vi "LIDAR V3 Mem1 Manager.vi"(0 "MeanFIFO":refnum<k21>="MeanVals1", 3 "StartAlgo":refnum<k21>="StartAlg2", 5 "MemRequest":refnum<k21>="MemRequest1", 6 "SignalMem":refnum<k21>="SignalMem1", 7 "MemDataAi":refnum<k21>="MemDataAi1", 8 "MemRequestDeb":refnum<k21>="MemRequestDeb1", 9 "MemDataDeb":refnum<k21>="MemDataDeb1", 10 "MemData":refnum<k21>="MemData1", 11 "Source Clk":refnum<k21>="100 MHz Clock") -> ()   [LabVIEW 2015]
uses:
  <vilib>/Platform/TimedLoop/XDataNode/timing_clust.ctl
  <vilib>/Platform/TimedLoop/XDataNode/nitl_modes.ctl
  <vilib>/Platform/TimedLoop/XDataNode/wakeup.ctl
  <vilib>/rvi/Emulation/niFpgaSctlEmulationGetInTimedLoop.vi
  <vilib>/rvi/Emulation/niFpgaEmulationReportErrorSimple.vi
  <vilib>/rvi/Emulation/niFpgaGetClockAttributes.vi
  <vilib>/rvi/Emulation/niFpgaCriticalErrorInLSC.vi
  <vilib>/rvi/DataTransferAndStorage/Container/Common/niFpgaContainerExecOnDevCompGetState.vi
  <vilib>/rvi/Emulation/niFpgaEmulationIsFPGAContextNoSignature.vi
  <vilib>/rvi/DataTransferAndStorage/Container/Common/niFpgaContainerGetUniqueNameForEmu.vi
  <vilib>/rvi/Emulation/niFpgaProcessEmulError.vi
  <vilib>/rvi/errors/nirviReportUnexpectedCaseInternalError (U32).vi
  <vilib>/rvi/Memory/Memory_Emulation/niFpgaMemoryEmulationCacheClearOnFirstRun.vi
  <vilib>/rvi/Memory/Memory_Emulation/nirvimemoryEmulationManagerCache_MakeExclusive.vi
  <vilib>/rvi/Memory/Memory_Emulation/niFpgaMemoryEmulationValidateCache.vi
  <vilib>/rvi/Memory/Memory_Emulation/nirvimemoryEmulationManagerCache_InsertValue.vi
  <vilib>/Utility/error.llb/Clear Errors.vi
  <vilib>/rvi/Memory/Memory_Emulation/nirvimemoryEmulationManagerCache_ReleaseExclusive.vi
  <vilib>/rvi/Memory/Memory_Emulation/nirvimemoryEmulationManagerCache_GetValue.vi
  <vilib>/rvi/Memory/Memory_Emulation/nirvimemoryEmulationManagerCache_SetValue.vi
  <vilib>/rvi/Emulation/niFpgaSctlEmulationResourceMgr.vi
  <vilib>/rvi/errors/niFpgaSetErrorForExecOnDevCompSimple.vi
  <vilib>/rvi/eio/common/nirviEmuReportErrorAndStop.vi
  <vilib>/rvi/FIFO/Fifo_Resource/nirvififoEmulationSetSize.vi
  <vilib>/rvi/FIFO/Fifo_Resource/nirviFifoEmulationQueueMgr.vi
  <instcachedir>/0/nirviFifoEmulationQueueMgr_E5CAEC123FF24DC58D834DCA3CDAA9B5.lvgen/nirviFifoEmulationQueueMgr_E5CAEC123FF24DC58D834DCA3CDAA9B5_002.vi
  <vilib>/rvi/FIFO/Fifo_Resource/nirvififoEmulationDetermineInputValidOut.vi
  <vilib>/rvi/FIFO/Fifo_Resource/nirvififoEmulationCreateLock.vi
  <vilib>/rvi/FIFO/Fifo_Resource/nirvififoEmulationObtainLock.vi
  <vilib>/rvi/FIFO/Fifo_Resource/nirvififoEmulationReleaseLock.vi
  <vilib>/rvi/occurrence/nirviWaitOnOccurrenceBase.vi
  <vilib>/rvi/errors/nirviReportUnexpectedCaseInternalError.vi
  <vilib>/rvi/interface/RandomDataEmulation/niFpgaRandomDataHandleErrors.vi
  <instcachedir>/0/nirviFifoEmulationQueueMgr_E5CAEC123FF24DC58D834DCA3CDAA9B5.lvgen/nirviFifoEmulationQueueMgr_E5CAEC123FF24DC58D834DCA3CDAA9B5_001.vi
  <vilib>/Platform/TimedLoop/XDataNode/XDataNode.xnode
  <vilib>/rvi/FXPMathLib/FxpAdd/XNode/nifxpmath_Add.xnode
  <vilib>/rvi/DataTransferAndStorage/Container/XNode/niFpgaContainer.xnode
  <vilib>/rvi/Memory/Memory_Emulation/niFpgaMemoryEmulationRefIn.vi
  <vilib>/rvi/FIFO/Fifo_Resource/niFpgaFifoEmulationRefIn.vi
  <vilib>/Platform/TimedLoop/XDataNode/XDNodeRunTimeDep.lvlib
  <vilib>/rvi/FXPMathLib/sim/FxpSim.dll
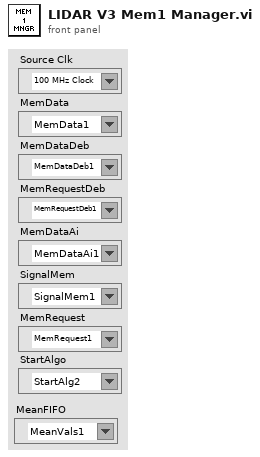
[diagram p1: front panel]
types:
  T1 = typedef "XDNodeRunTimeDep.lvlib/timing_clust.ctl" = cluster{"Expected End [f-1]":u64, "Actual End [f-1]":u64, "Finished Late? [f-1]":bool, "Expected End [i-1]":u64, "Actual End [i-1]":u64, "Finished Late? [i-1]":bool, "Expected Start [i]":u64, "Actual Start [i]":u64, "Expected Start [f]":u64, "Actual Start [f]":u64, "Source Name":string, "Structure Name":string, "Period":i64, "Deadline":i64, "Offset":i64, "Start":i64, "Priority":i32, "Timeout":i32, "Mode":T2, "Wakeup Reason":T3, "Error":errorcluster, "Source Type":string, "Secondary Source Type":string, "Global End Time":u64, "Global Start Time":u64, "Frame Duration":u64, "Iteration Duration":u64, "Assigned CPU":i32, "I/O Scan Engine Mode":u32}
  T2 = typedef "XDNodeRunTimeDep.lvlib/nitl_modes.ctl" = enum32{"No Change", "Process missed periods, maintain original phase", "Discard missed periods, maintain original phase", "Process missed periods, ignore original phase", "Discard missed periods, ignore original phase"}
  T3 = typedef "XDNodeRunTimeDep.lvlib/wakeup.ctl" = enum32{"Normal", "Aborted", "Asynchronous wakeup", "Timing source error", "Timed loop error", "Timeout"}
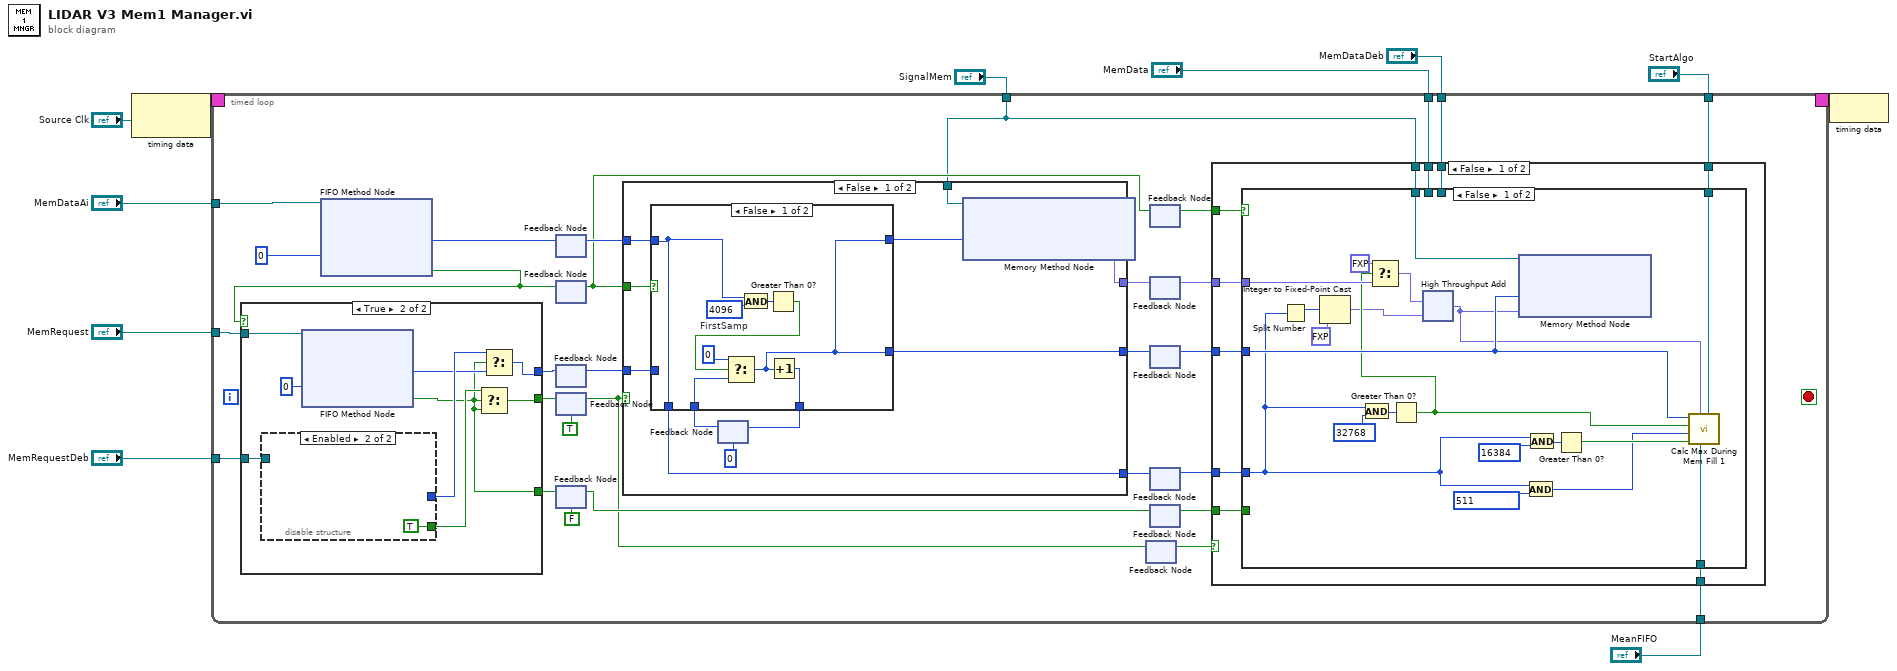
[diagram p0: block diagram]
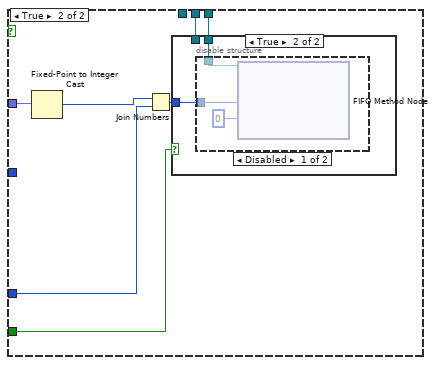
[diagram p2: hidden frame]
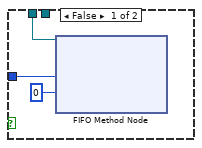
[diagram p3: hidden frame]
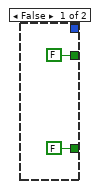
[diagram p8: hidden frame]
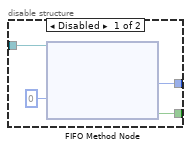
[diagram p9: hidden frame]
diagram:
  n1 = node-c288("Source Clk") -> (w11:T1)
  n2 = timed-loop {
    timing: w11 -> [_]
    timing-out: [_] -> w10
    tunnel: "MemDataAi" -> [w29]
    tunnel: "MemRequest" -> [w28]
    tunnel: "MemRequestDeb" -> [w27]
    tunnel: "SignalMem" -> [w26]
    tunnel: "MemData" -> [w25]
    tunnel: "MemDataDeb" -> [w24]
    tunnel: "MeanFIFO" -> [w13]
    tunnel: "StartAlgo" -> [w12]
    stop <- _ stop-if-true
    n3 = xnode ("FIFO Method Node")("Timeout"=0, "FIFO In"=w29) -> ("Element"=w41:u32, "Timed Out?"=w38:bool)  [unwired: 1 out]
    n4 = case shown="True" w38 {
      tunnel: [FALSE ("Timed Out?") w116] -> w39
      tunnel: [_ w113] -> w37
      tunnel: [FALSE ("Timed Out?") w112] -> w32
      tunnel: w28 -> [_ w111]
      tunnel: w27 -> [_ w110]
      frame False {
      }
      frame True {
        n5 = disable-structure shown="Enabled" {
          disable-tunnel: [w121 TRUE ("Timed Out?")] -> w117
          disable-tunnel: [w120 _] -> w115
          disable-tunnel: w110 -> [w119 _]
          frame Disabled {
            n6 = xnode ("FIFO Method Node")("Timeout"=0, "FIFO In"=w119) -> ("Element"=w120:u32, "Timed Out?"=w121:bool)  [unwired: 1 out]
          }
          frame Enabled {
          }
        }
        n7 = xnode ("FIFO Method Node")("Timeout"=0, "FIFO In"=w111) -> ("Element"=w114:u32, "Timed Out?"=w112:bool)  [unwired: 1 out]
        n8 = Select(t=w117, s=w112, f=w112) -> (s? t:f=w116:bool)
        n9 = Select(t=w115, s=w112, f=w114) -> (s? t:f=w113:u32)
      }
    }
    n10 = feedback-in #1(w41) -> ()
    n11 = feedback #1() -> (w36:u32)  [unwired: 1 in]
    n12 = feedback-in #2(w38) -> ()
    n13 = feedback #2() -> (w35:bool)  [unwired: 1 in]
    n14 = feedback-in #3(w37) -> ()
    n15 = feedback #3() -> (w34:u32)  [unwired: 1 in]
    n16 = feedback-in #4(w39) -> ()
    n17 = feedback #4(TRUE ("Timed Out?")) -> (w15:bool)
    n18 = feedback-in #5(w32) -> ()
    n19 = feedback #5(FALSE ("Timed Out?")) -> (w33:bool)
    n20 = case shown="False" w15 {
      tunnel: w36 -> [w97 _]
      tunnel: w35 -> [w96 _]
      tunnel: w34 -> [w95 _]
      tunnel: w26 -> [w94 _]
      tunnel: [w93 _] -> w23
      tunnel: [w91 _] -> w22
      tunnel: [w87 _] -> w21
      frame False {
        n21 = feedback #6(u32 0 ("Element")) -> (w88:u32)
        n22 = case shown="False" w96 {
          tunnel: w97 -> [w104 _]
          tunnel: [w98 w107] -> w92
          tunnel: w95 -> [_ w107]
          tunnel: [w104 w107] -> w91
          tunnel: [w99 w106] -> w89
          tunnel: w88 -> [w100 w106]
          tunnel: [w98 w106] -> w87
          frame False {
            w105 = u32 4096  # FirstSamp
            n23 = And(x=w104, y=w105) -> (x .and. y?=w103:u32)
            n24 = Greater Than 0?(x=w103) -> (x > 0?=w102:bool)
            n25 = Select(t=u32 0 ("Element"), s=w102, f=w100) -> (s? t:f=w98:u32)
            n26 = Increment(x=w98) -> (x+1=w99:u32)
          }
          frame True {
          }
        }
        n27 = feedback-in #6(w89) -> ()
        n28 = xnode ("Memory Method Node")("Address"=w92, "Memory In"=w94) -> ("Data"=w93:fxp<+/-,22,22>)  [unwired: 1 out]
      }
      frame True {
      }
    }
    n29 = feedback-in #7(w15) -> ()
    n30 = feedback #7() -> (w14:bool)  [unwired: 1 in]
    n31 = feedback-in #8(w35) -> ()
    n32 = feedback #8() -> (w20:bool)  [unwired: 1 in]
    n33 = feedback-in #9(w23) -> ()
    n34 = feedback #9() -> (w19:fxp<+/-,22,22>)  [unwired: 1 in]
    n35 = feedback-in #10(w21) -> ()
    n36 = feedback #10() -> (w18:u32)  [unwired: 1 in]
    n37 = feedback-in #11(w22) -> ()
    n38 = feedback #11() -> (w17:u32)  [unwired: 1 in]
    n39 = feedback-in #12(w33) -> ()
    n40 = feedback #12() -> (w16:bool)  [unwired: 1 in]
    n41 = case shown="False" w14 {
      tunnel: w26 -> [w51 _]
      tunnel: w25 -> [w50 _]
      tunnel: w24 -> [w49 _]
      tunnel: w20 -> [w48 _]
      tunnel: w19 -> [w47 _]
      tunnel: w18 -> [w46 _]
      tunnel: w17 -> [w45 _]
      tunnel: w16 -> [w44 _]
      tunnel: w13 -> [w43 _]
      tunnel: w12 -> [w42 _]
      frame False {
        n42 = case shown="False" w48 {
          tunnel: w47 -> [w70 w78]
          tunnel: w45 -> [w55 w75]
          tunnel: w44 -> [_ w74]
          tunnel: w46 -> [w64 _]
          tunnel: w51 -> [w61 _]
          tunnel: w50 -> [_ w73]
          tunnel: w49 -> [_ w72]
          tunnel: w43 -> [w53 _]
          tunnel: w42 -> [w52 _]
          frame False {
            n43 = Split Number(x=w55) -> (hi(x)=w56:u16)  [unwired: 1 out]
            n44 = Integer to Fixed-Point Cast(fixed-point type=fxp<+/-,16,16> 0.0, integer=w56) -> (fixed-point=w54:fxp<+/-,16,16>)
            n45 = And(x=w55, y=u32 32768) -> (x .and. y?=w59:u32)
            n46 = Greater Than 0?(x=w59) -> (x > 0?=w58:bool)
            n47 = Select(t=fxp<+/-,22,22> 0.0, s=w58, f=w70) -> (s? t:f=w69:fxp<+/-,22,22>)
            n48 = xnode ("High Throughput Add")("x"=w69, "y"=w54) -> ("x+y"=w63:fxp<+/-,22,22>)
            n49 = xnode ("Memory Method Node")("Address"=w64, "Data"=w63, "Memory In"=w61) -> ()  [unwired: 1 out]
            n50 = And(x=w55, y=u32 511) -> (x .and. y?=w62:u32)
            n51 = And(x=w55, y=u32 16384) -> (x .and. y?=w66:u32)
            n52 = Greater Than 0?(x=w66) -> (x > 0?=w68:bool)
            n53 = call "Calc Max During Mem Fill 1.vi"("StartAlgo"=w52, "MeanFIFO"=w53, "Value"=w63, "LastIterration"=w68, "ActiveLedIndex"=w62, "FirstIterration"=w58, "Address"=w64) -> ()  [unwired: 5 in]
          }
          frame True {
            n54 = Fixed-Point to Integer Cast(1:w78) -> (0:w76:i32)
            n55 = Join Numbers(hi=w76, lo=w75) -> ((hi.lo)=w77:u64)
            n56 = case shown="False" w74 {
              tunnel: w77 -> [w80 w83]
              tunnel: w73 -> [w79 _]
              tunnel: w72 -> [_ w82]
              frame False {
                n57 = xnode ("FIFO Method Node")("Element"=w80, "Timeout"=0, "FIFO In"=w79) -> ()  [unwired: 2 out]
              }
              frame True {
                n58 = disable-structure shown="Disabled" {
                  disable-tunnel: w83 -> [w85 _]
                  disable-tunnel: w82 -> [w84 _]
                  frame Disabled {
                    n59 = xnode ("FIFO Method Node")("Element"=w85, "Timeout"=0, "FIFO In"=w84) -> ()  [unwired: 2 out]
                  }
                  frame Enabled {
                  }
                }
              }
            }
          }
        }
      }
      frame True {
      }
    }
  }
  n60 = node-c288(w10) -> ()
